vi "Average tau0.vi"(4 "filter changed?":bool, 6 "filter":bool, 8 "error in":errorcluster, 9 "# of shots":i32, 11 "CRDS Cell in":refnum<class "CRDS Cell.lvclass">) -> (0 "error out":errorcluster, 3 "CRDS Cell out":refnum<class "CRDS Cell.lvclass">)   [LabVIEW 2015, in "CRDS Cell.lvclass"]
doc: "Average taus recorded on filter to give a mean tau0. The values tau0 and tau0cor will be averaged over the number of times this vi is called or the value of <b># of shots</b>, whichever is smaller.\n\nOnly accessors can throw errors here."
uses:
  CRDS Cell.lvclass
  CRDS Cell.lvclass/CRDS Cell.ctl
  Data/Cell/CRDS Cell Data.lvclass/CRDS Cell Data.ctl
  <vilib>/Analysis/baseanly.llb/Mean (DBL).vi
  Read Data.vi
  Data/Cell/Write extParam.vi
  Write Data.vi
  Data/Cell/Read extParam.vi
  Write corr tau0.vi
  Write tau_0.vi
  Data/Cell/CRDS Cell Data.lvclass
  <vilib>/Analysis/NI_AALBase.lvlib
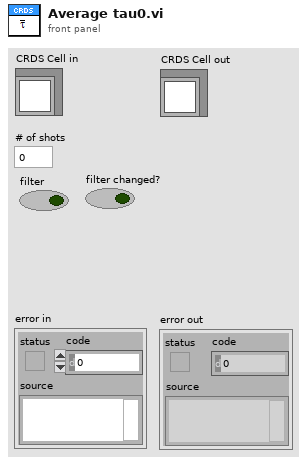
[diagram p1: front panel]
types:
  T1 = typedef "extparam.ctl" = cluster{"Tau":sgl, "Tau0cor":sgl, "ext":sgl, "extCorr":sgl, "stdevTau":sgl, "eTau":sgl, "taucorr":sgl, "Tau0":sgl, "max":sgl}
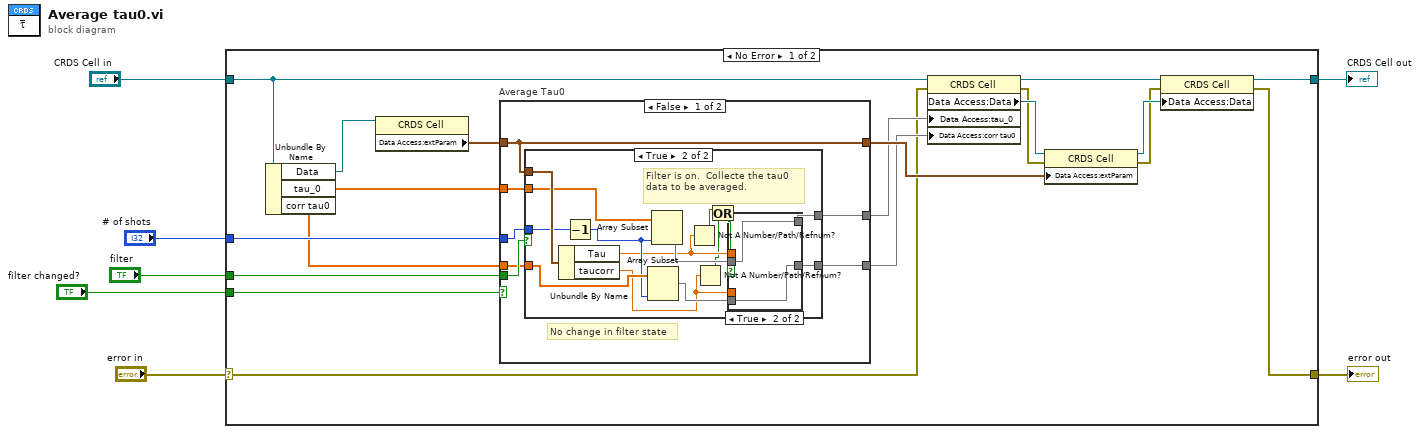
[diagram p0: block diagram]
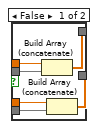
[diagram p3: hidden frame]
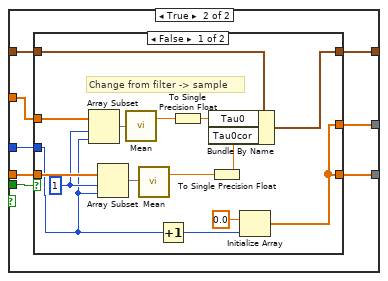
[diagram p4: hidden frame]
diagram:
  n1 = case shown="No Error" "error in" {
    selector: "error in" -> [w15 w85]
    tunnel: [w12 w85] -> w6
    tunnel: [w20 w84] -> w4
    tunnel: "CRDS Cell in" -> [w10 w84]
    tunnel: "# of shots" -> [w26 _]
    tunnel: "filter" -> [w25 _]
    tunnel: "filter changed?" -> [w11 _]
    frame No Error {
      n2 = Unbundle By Name(w10) -> ("Data"=w8:refnum<class "CRDS Cell Data.lvclass">, "tau_0"=w19:dbl[], "corr tau0"=w18:dbl[])
      n3 = property class="CRDS Cell"(reference=w8) -> ("Data Access:extParam"=w9:T1)  [unwired: 1 in, 2 out]
      n4 = case "Average Tau0" shown="False" w11 {
        tunnel: w25 -> [w30 w65]
        tunnel: w9 -> [w33 w64]
        tunnel: [w33 w63] -> w23
        tunnel: w19 -> [w32 w62]
        tunnel: [w31 w61] -> w16
        tunnel: w18 -> [w29 w60]
        tunnel: [w28 w59] -> w17
        tunnel: w26 -> [w27 w58]
        frame False {
          # "No change in filter state"
          n5 = case shown="True" w30 {
            tunnel: w33 -> [_ w49]
            tunnel: w32 -> [w35 w46]
            tunnel: [w35 w48] -> w31
            tunnel: w29 -> [w34 w44]
            tunnel: [w34 w41] -> w28
            tunnel: w27 -> [_ w47]
            frame False {
              # "On sample."
            }
            frame True {
              # "Filter is on.  Collecte the tau0  data to be averaged."
              n6 = Unbundle By Name(w49) -> ("Tau"=w40:sgl, "taucorr"=w39:sgl)
              n7 = Decrement(x=w47) -> (x-1=w43:i32)
              n8 = Array Subset(array=w44, length=w43) -> (w42:dbl[])  [unwired: 1 in]
              n9 = Array Subset(array=w46, length=w43) -> (w45:dbl[])  [unwired: 1 in]
              n10 = Not A Number/Path/Refnum?(number/path/refnum=w40) -> (NaN/Path/Refnum?=w38:bool)
              n11 = Not A Number/Path/Refnum?(number/path/refnum=w39) -> (NaN/Path/Refnum?=w37:bool)
              n12 = Or(x=w38, y=w37) -> (x .or. y?=w36:bool)
              n13 = case shown="True" w36 {
                tunnel: w40 -> [w55 _]
                tunnel: [w54 w57] -> w48
                tunnel: w45 -> [w53 w57]
                tunnel: w42 -> [w52 w56]
                tunnel: w39 -> [w51 _]
                tunnel: [w50 w56] -> w41
                frame False {
                  n14 = Build Array (concatenate)(w55, w53) -> (w54:dbl[])
                  n15 = Build Array (concatenate)(w51, w52) -> (w50:dbl[])
                }
                frame True {
                }
              }
            }
          }
        }
        frame True {
          n16 = case shown="False" w65 {
            tunnel: w64 -> [w80 w83]
            tunnel: [w79 w83] -> w63
            tunnel: w62 -> [w71 w82]
            tunnel: [w73 w82] -> w61
            tunnel: w60 -> [w70 w81]
            tunnel: [w73 w81] -> w59
            tunnel: w58 -> [w68 _]
            frame False {
              w69 = 1 ("index")
              # "Change from filter -> sample"
              n17 = Array Subset(array=w71, index=w69, length=w68) -> (w67:dbl[])
              n18 = Array Subset(array=w70, index=w69, length=w68) -> (w66:dbl[])
              n19 = call-poly <vilib>:"Mean.vi"("X"=w67) -> ("mean"=w78:dbl)  [unwired: 1 out]
              n20 = call-poly <vilib>:"Mean.vi"("X"=w66) -> ("mean"=w76:dbl)  [unwired: 1 out]
              n21 = Increment(x=w68) -> (x+1=w72:i32)
              n22 = To Single Precision Float(number=w78) -> (single precision float=w77:sgl)
              n23 = To Single Precision Float(number=w76) -> (single precision float=w75:sgl)
              n24 = Bundle By Name(cluster=w80, "Tau0"=w77, "Tau0cor"=w75) -> (w79:T1)
              n25 = Initialize Array(0.0, w72) -> (w73:dbl[])
            }
            frame True {
              # "Change from sample -> filter. Do nothing, the matrices have already been zeroed."
            }
          }
        }
      }
      n26 = property class="CRDS Cell"(reference=w10, error in=w15, "Data Access:tau_0"=w16, "Data Access:corr tau0"=w17) -> (reference out=w22:refnum<class "CRDS Cell.lvclass">, error out=w14:errorcluster, "Data Access:Data"=w24:refnum<class "CRDS Cell Data.lvclass">)
      n27 = property class="CRDS Cell"(reference=w24, error in=w14, "Data Access:extParam"=w23) -> (reference out=w21:refnum<class "CRDS Cell Data.lvclass">, error out=w13:errorcluster)
      n28 = property class="CRDS Cell"(reference=w22, error in=w13, "Data Access:Data"=w21) -> (reference out=w20:refnum<class "CRDS Cell.lvclass">, error out=w12:errorcluster)
    }
    frame Error {
    }
  }
  "error out" <- w6
  "CRDS Cell out" <- w4
